vi "CoilsClose.vi"(8 "error in":errorcluster, 9 "Coils DO Task in":refnum<k21>, 10 "Coils AO Task in":refnum<k21>, 11 "Keithley USB":refnum<visa-resource-name>) -> (0 "error out":errorcluster)   [LabVIEW 2012]
uses:
  Keithley KE22xx Series/Keithley KE22xx Series.lvlib
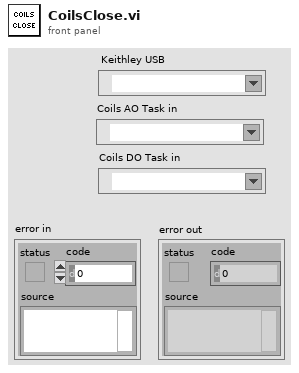
[diagram p1: front panel]
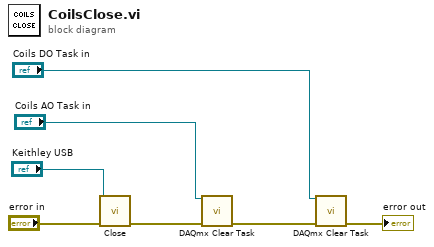
[diagram p0: block diagram]
diagram:
  n1 = call "Close.vi"("error in (no error)"="error in", "VISA resource name"="Keithley USB") -> ("error out"=w7:errorcluster)  [unwired: 9 in]
  n2 = call <vilib>:"DAQmx Clear Task.vi"("task in"="Coils AO Task in", "error in"=w7) -> ("error out"=w6:errorcluster)  [unwired: 13 in]
  n3 = call <vilib>:"DAQmx Clear Task.vi"("task in"="Coils DO Task in", "error in"=w6) -> ("error out"=→"error out":errorcluster)  [unwired: 13 in]
